vi "Node - Get Local Ch Data.vi"(8 "error in (no error)":errorcluster) -> (0 "error out":errorcluster)   [LabVIEW 2016]
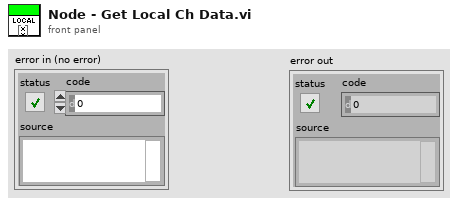
[diagram p1: front panel]
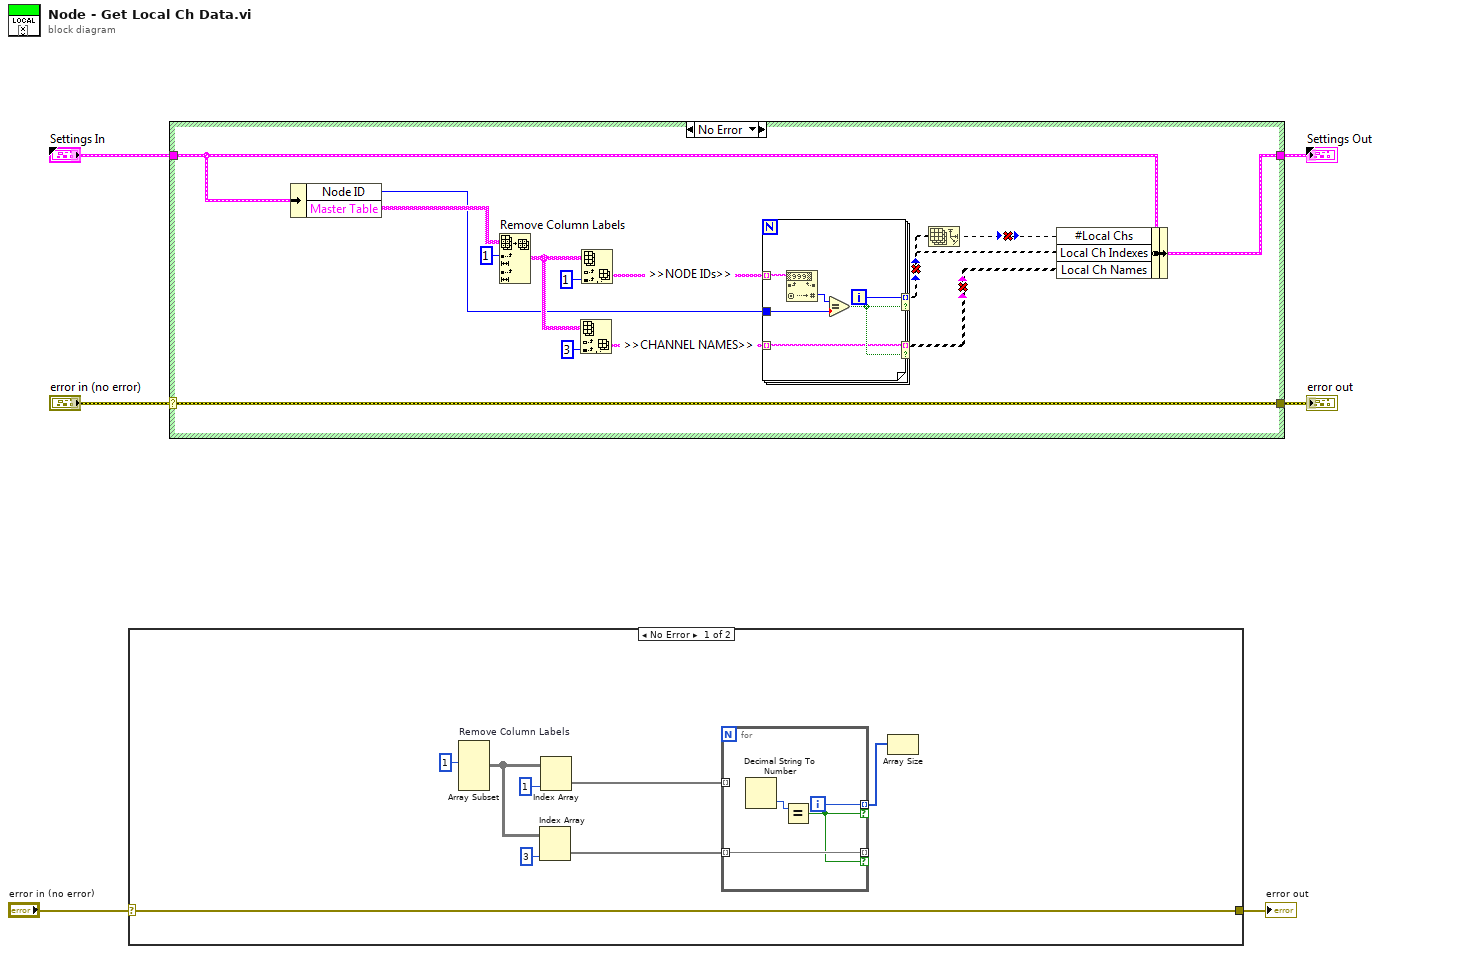
[diagram p0: block diagram]
diagram:
  n1 = case shown="No Error" "error in (no error)" {
    selector: "error in (no error)" -> [w9 w15]
    tunnel: [w9 w15] -> w1
    frame No Error {
      n2 = Array Subset "Remove Column Labels"(index (row)=1 ("index")) -> (w5:void[][])  [unwired: 4 in]
      n3 = Index Array(array=w5, index (col)=3 ("disabled index (col)")) -> (element=w4:void[])  [unwired: 1 in]
      n4 = Index Array(array=w5, index (col)=1 ("index (row)")) -> (element=w7:void[])  [unwired: 1 in]
      n5 = for {
        tunnel: w7 -> [_] mode=indexing
        tunnel: [w13] -> w3 mode=indexing if=w11
        tunnel: w4 -> [w12] mode=indexing
        tunnel: [w12] -> _ mode=indexing if=w11
        i -> [w13]
        n6 = Decimal String To Number() -> (number=w14:i32)  [unwired: 3 in, 1 out]
        n7 = Equal?(x=w14) -> (x = y?=w11:bool)  [unwired: 1 in]
      }
      n8 = Array Size(array=w3) -> ()  [unwired: 1 out]
    }
    frame Error {
    }
  }
  "error out" <- w1
